vi "Subheader.vi"(8 "error in (no error)":errorcluster, 11 "Mitsubishi PLC in":refnum<class "Mitsubishi PLC.lvclass">) -> (0 "error out":errorcluster, 3 "Mitsubishi PLC out":refnum<class "Mitsubishi PLC.lvclass">)   [LabVIEW 2019, in "Mitsubishi PLC.lvclass"]
uses:
  Mitsubishi PLC.lvclass
  Mitsubishi PLC.lvclass/Mitsubishi PLC.ctl
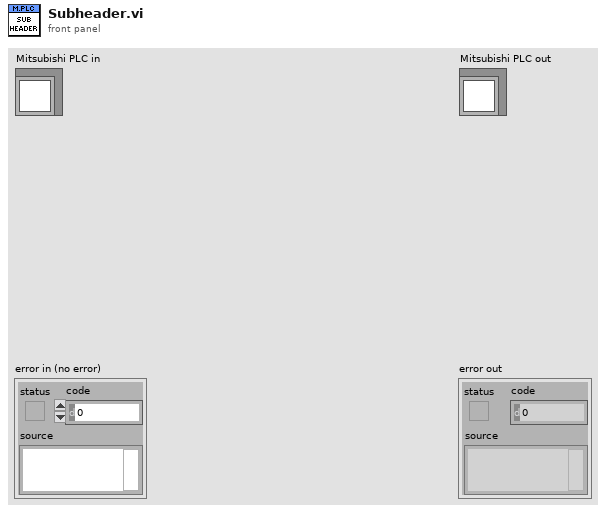
[diagram p1: front panel]
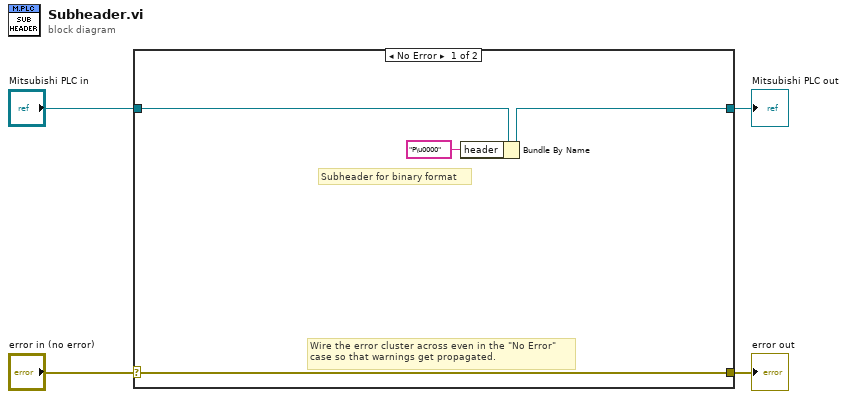
[diagram p0: block diagram]
diagram:
  n1 = case shown="No Error" "error in (no error)" {
    selector: "error in (no error)" -> [w7 w10]
    tunnel: [w7 w10] -> w3
    tunnel: [w6 w9] -> w1
    tunnel: "Mitsubishi PLC in" -> [w8 w9]
    frame No Error {
      # "Subheader for binary format"
      # "Wire the error cluster across even in the \"No Error\"\ncase so that warnings get propagated."
      n2 = Bundle By Name(cluster=w8, "header"="P\u0000") -> (w6:refnum<class "Mitsubishi PLC.lvclass">)
    }
    frame Error {
    }
  }
  "error out" <- w3
  "Mitsubishi PLC out" <- w1
